vi "Query Arbitrary Waveform.vi"(8 "error in (no error)":errorcluster, 10 "Waveform Slot (1: Slot 1)":i32(ring)=1 items=["Slot 1"=1, "Slot 2"=2, "Slot 3"=3, "Slot 4"=4], 11 "VISA resource name":refnum<visa-resource-name>) -> (0 "error out":errorcluster, 1 "Waveform Time":string, 2 "Waveform Date":string, 3 "VISA resource name out":refnum<visa-resource-name>)   [LabVIEW 2017, in "Scope.lvlib" / "Tektronix DPO MSO 2000 4000 Series.lvlib"]
doc: "Queries the date and time of the specified arbitrary waveform slot.\n\n<B>Notes:</B>\n(1) This VI is available for MDO3000 Series only.\n\n(2) Requires the MDO3AFG option to be installed."
uses:
  Tektronix DPO MSO 2000 4000 Series.lvlib
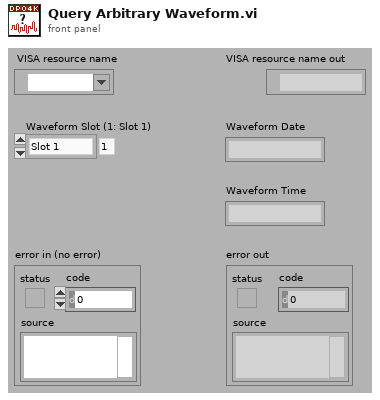
[diagram p1: front panel]
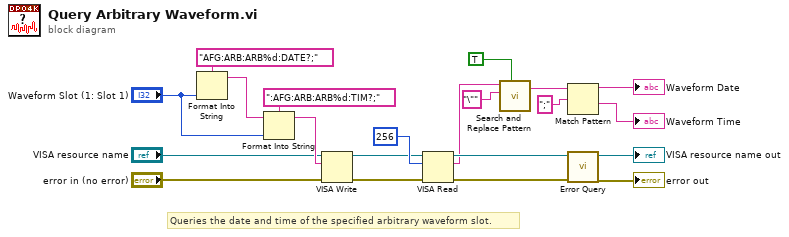
[diagram p0: block diagram]
diagram:
  # "Queries the date and time of the specified arbitrary waveform slot."
  n1 = Format Into String(format string="AFG:ARB:ARB%d:DATE?;", "Waveform Slot (1: Slot 1)") -> (resulting string=w18:string)  [unwired: 2 in, 1 out]
  n2 = Format Into String(format string=":AFG:ARB:ARB%d:TIM?;", initial string=w18, "Waveform Slot (1: Slot 1)") -> (resulting string=w17:string)  [unwired: 1 in, 1 out]
  n3 = VISA Write(VISA resource name="VISA resource name", write buffer=w17, error in (no error)="error in (no error)") -> (VISA resource name out=w11:refnum<visa-resource-name>, error out=w10:errorcluster)  [unwired: 1 out]
  n4 = VISA Read(VISA resource name=w11, byte count=u32 256, error in (no error)=w10) -> (VISA resource name out=w9:refnum<visa-resource-name>, read buffer=w4:string, error out=w8:errorcluster)  [unwired: 1 out]
  n5 = call <vilib>:"Search and Replace Pattern.vi"("string"=w4, "regular expression (\"\")"="\"" ("regular expression (\"\")"), "replace all? (F)"=TRUE) -> ("result string"=w3:string)  [unwired: 2 in, 1 out]
  n6 = Match Pattern(string=w3, regular expression=";") -> (before substring=→"Waveform Date":string, after substring=→"Waveform Time":string)  [unwired: 1 in, 2 out]
  n7 = call "Error Query.vi"("error in (no error)"=w8, "VISA resource name"=w9) -> ("error out"=→"error out":errorcluster, "VISA resource name out"=→"VISA resource name out":refnum<visa-resource-name>)  [unwired: 6 in, 2 out]
